vi "Relay_EOL_FCT.vi"(9 "FCT/EOL":i32, 10 "EOL_Relay - OUTPUT":T3, 11 "FCT_Relay - OUTPUT":T2) -> (3 "output cluster":cluster{cluster{bool, "OUTPUT_CH_Relay":T1}[]})   [LabVIEW 2024]
uses:
  Modules/MANUAL_MODE/support/EOL_DO_UI.ctl
  Modules/MANUAL_MODE/support/FCT_DO_UI.ctl
  Modules/Relay_Module/support/Relay_Enum_OUT.ctl
  Modules/Relay_Module/Relay_Module.lvlib
panel:
  in  "Relay-FCT/EOL":enum32{"FCT", "EOL"}(tab)
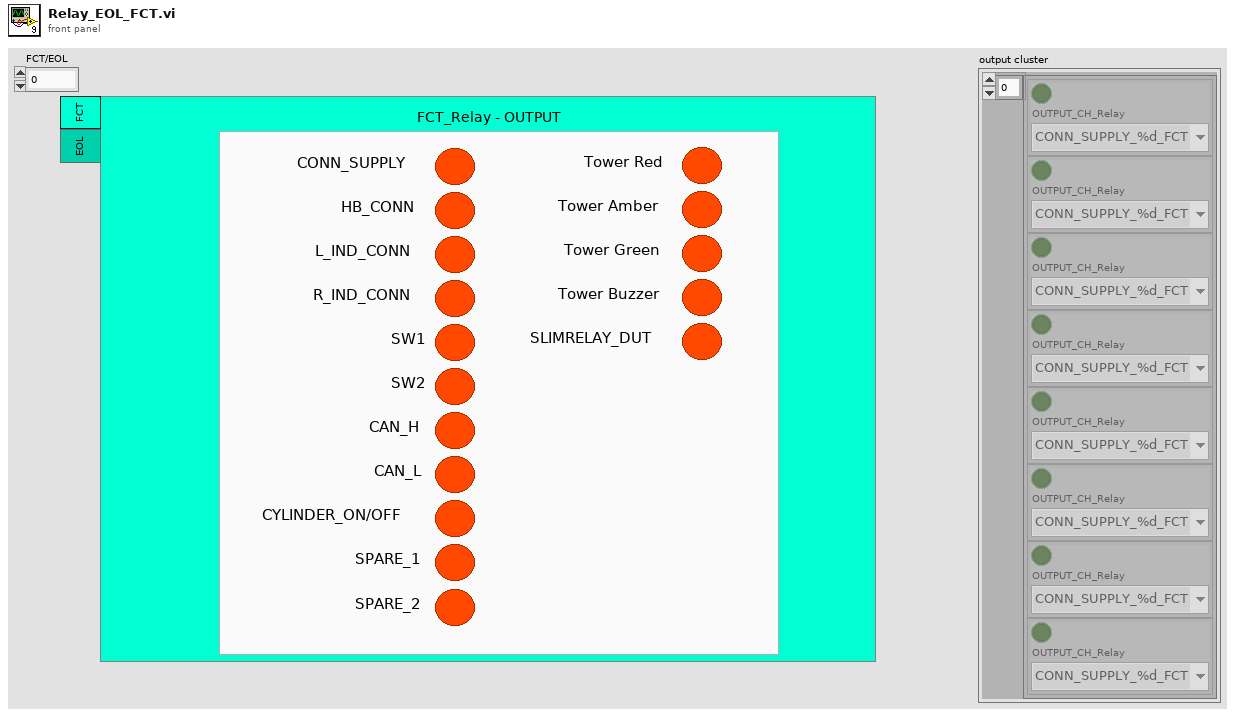
[diagram p1: front panel]
types:
  T1 = typedef "Relay_Module.lvlib/Relay_Enum_OUT.ctl" = enum16{"CONN_SUPPLY_%d_FCT", "HB_CONN_%d_FCT", "L_IND_CONN_%d_FCT", "R_IND_CONN_%d_FCT", "SW1_%d_FCT", "SW2_%d_FCT", "CAN_H_%d_FCT", "CAN_L_%d_FCT", "CYLINDER_ON/OFF_%d_FCT", "SPARE_1_%d_FCT", "SPARE_2_%d_FCT", "Tower Red", "Tower Amber", "Tower Green", "Tower Buzzer", "SLIMRELAY_DUT_%d_FCT", "GND_DMM_%d_EOL", "CAN_H_RES_%d_EOL", "CAN_L_RES_%d_EOL", "L_IND_RES_%d_EOL", "R_IND_RES_%d_EOL", "HB_CONN_DMM_%d_EOL", "14V_RES_%d_EOL", "CAN_L_(DMM-)_%d_EOL", "CAN_H_%d_EOL", "CAN_L_%d_EOL", "14V_%d_EOL", "GND_%d_EOL", "HB_CONN_%d_EOL", "L_IND_%d_EOL", "R_IND_%d_EOL", "CYLINDER_DUT_%d_EOL", "CYL_PB_1_%d_EOL", "CYL_PB_2_%d_EOL", "DUT_PASS_%d_EOL", "DUT_FAIL_%d_EOL", "SPARE1_%d_EOL", "Tower Red_EOL", "Tower Amber_EOL", "Tower Green_EOL", "Tower Buzzer_EOL"}
  T2 = typedef "FCT_DO_UI.ctl" = cluster{"CONN_SUPPLY":bool, "HB_CONN":bool, "L_IND_CONN":bool, "R_IND_CONN":bool, "SW1":bool, "SW2":bool, "CAN_H":bool, "CAN_L":bool, "CYLINDER_ON/OFF":bool, "SPARE_1":bool, "SPARE_2":bool, "Tower Red":bool, "Tower Amber":bool, "Tower Green":bool, "Tower Buzzer":bool, "SLIMRELAY_DUT":bool}
  T3 = typedef "EOL_DO_UI.ctl" = cluster{"GND_DMM":bool, "CAN_H_RES":bool, "CAN_L_RES":bool, "L_IND_RES":bool, "R_IND_RES":bool, "HB_CONN_DMM":bool, "14V_RES":bool, "CAN_L_(DMM-)":bool, "CAN_H":bool, "CAN_L":bool, "14V":bool, "GND":bool, "HB_CONN":bool, "L_IND":bool, "R_IND":bool, "CYLINDER_DUT":bool, "CYL_PB_1":bool, "CYL_PB_2":bool, "DUT_PASS":bool, "DUT_FAIL":bool, "SPARE1":bool, "Tower Red_EOL":bool, "Tower Amber_EOL":bool, "Tower Green_EOL":bool, "Tower Buzzer_EOL":bool}
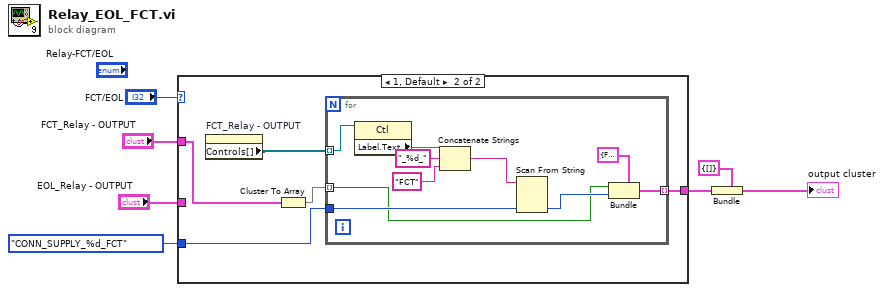
[diagram p0: block diagram]
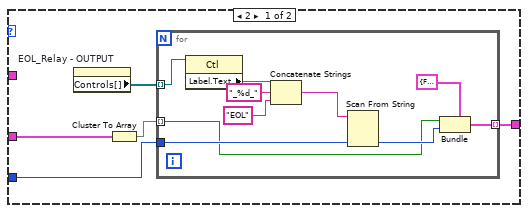
[diagram p2: hidden frame]
diagram:
  n1 = case shown="1, Default" "FCT/EOL" {
    tunnel: "FCT_Relay - OUTPUT" -> [_ w23]
    tunnel: "EOL_Relay - OUTPUT" -> [w12 _]
    tunnel: Relay_Enum_OUT."CONN_SUPPLY_%d_FCT" ("OUTPUT_CH_Relay") -> [w10 w26]
    tunnel: [w8 w25] -> w4
    frame 2 {
      n2 = property on="EOL_Relay - OUTPUT" class="Clust (strict)"() -> ("Controls[]"=w9:refnum<vi>[])  [unwired: 2 in, 2 out]
      n3 = Cluster To Array(cluster=w12) -> (array=w11:bool[])
      n4 = for {
        tunnel: w11 -> [w13] mode=indexing
        tunnel: w10 -> [w22]
        tunnel: w9 -> [w21] mode=indexing
        tunnel: [w16] -> w8 mode=indexing
        n5 = property class="Ctl"(reference=w21) -> ("Label.Text"=w20:string)  [unwired: 1 in, 2 out]
        n6 = Concatenate Strings(w20, "_%d_" ("string"), "EOL" ("string")) -> (w17:string)
        n7 = Scan From String(input string=w17, default 1=w22) -> (output 1=w14:T1)  [unwired: 3 in, 3 out]
        n8 = Bundle(cluster=cluster{bool, "OUTPUT_CH_Relay":T1} {FALSE, "OUTPUT_CH_Relay"=enum."CONN_SUPPLY_%d_FCT"}, w13, "OUTPUT_CH_Relay"=w14) -> (w16:cluster{bool, "OUTPUT_CH_Relay":T1})
      }
    }
    frame 1, Default {
      n9 = property on="FCT_Relay - OUTPUT" class="Clust (strict)"() -> ("Controls[]"=w24:refnum<vi>[])  [unwired: 2 in, 2 out]
      n10 = Cluster To Array(cluster=w23) -> (array=w27:bool[])
      n11 = for {
        tunnel: w27 -> [w28] mode=indexing
        tunnel: w26 -> [w37]
        tunnel: w24 -> [w36] mode=indexing
        tunnel: [w30] -> w25 mode=indexing
        n12 = property class="Ctl"(reference=w36) -> ("Label.Text"=w35:string)  [unwired: 1 in, 2 out]
        n13 = Concatenate Strings(w35, "_%d_" ("string"), "FCT" ("string")) -> (w32:string)
        n14 = Scan From String(input string=w32, default 1=w37) -> (output 1=w29:T1)  [unwired: 3 in, 3 out]
        n15 = Bundle(cluster=cluster{bool, "OUTPUT_CH_Relay":T1} {FALSE, "OUTPUT_CH_Relay"=enum."CONN_SUPPLY_%d_FCT"}, w28, "OUTPUT_CH_Relay"=w29) -> (w30:cluster{bool, "OUTPUT_CH_Relay":T1})
      }
    }
  }
  n16 = Bundle(cluster=cluster{cluster{bool, "OUTPUT_CH_Relay":T1}[]} {[]}, w4) -> (→"output cluster":cluster{cluster{bool, "OUTPUT_CH_Relay":T1}[]})
